vi "DSF.Engine.Memory.Cache.Get Transfers Group.vi"(10 "Transfer Group id":i32, 11 "Cache in":refnum<class "DSF.Engine.Memory.Cache.lvclass">) -> (2 "Transfers Group":refnum<class "DSF.Engine.Transfer Group.lvclass">, 3 "Cache out":refnum<class "DSF.Engine.Memory.Cache.lvclass">)   [LabVIEW 2017, in "DSF.Engine.lvlib" / "DSF.Engine.Memory.Cache.lvclass"]
uses:
  DSF.Engine.Memory.Cache.lvclass
  Transfer/DSF.Engine.Transfer Group.lvclass
  DSF.Engine.Memory.Cache.lvclass/DSF.Engine.Memory.Cache.ctl
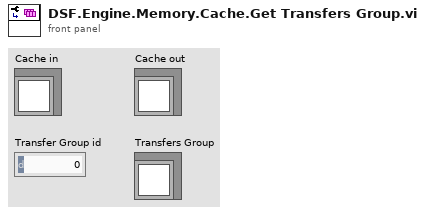
[diagram p1: front panel]
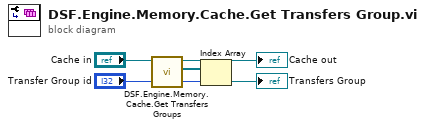
[diagram p0: block diagram]
diagram:
  n1 = call "DSF.Engine.Memory.Cache.Get Transfers Groups.vi"("Cache in"="Cache in") -> ("Transfers Groups"=w3:refnum<class "DSF.Engine.Transfer Group.lvclass">[], "Cache out"=→"Cache out":refnum<class "DSF.Engine.Memory.Cache.lvclass">)  [unwired: 9 in]
  n2 = Index Array(array=w3, index="Transfer Group id") -> (element=→"Transfers Group":refnum<class "DSF.Engine.Transfer Group.lvclass">)
